vi "运维调试_总磷.vi"() -> ()   [LabVIEW 2016, in "斯坦道总磷.lvlib"]
uses:
  <vilib>/Utility/miscctls.llb/LVPointTypeDef.ctl
  <vilib>/Utility/config.llb/NI_LVConfig.lvlib
  <vilib>/ptbypt/NI_PtbyPt.lvlib
panel:
  out "二级权限":bool
  out "一级权限":bool
  out "输入密码":u32
  out "权限锁":bool
  in  "流程固件":bool
  in  "仪器参数设置":bool
  in  "量程参数读取":T1
  in  "模块启用":bool
  in  "串口设置":bool
  in  "公式一键写入":bool
  in  "流程路径":path=path "C:/Users/STD/Documents/斯坦道流程文件/流程.xml"
  in  "曲线模型":cluster{"X^2":dbl, "X":dbl, "B":dbl}(xcontrol)
  out "字符串":string
  in  "质控参数设置":bool
  in  "总磷自动测试量程配置":T2
  out "温度2":sgl
  out "温度1":sgl
  out "ADC":sgl
  out "固件版本号":string
  in  "数组":string[](array[string])
  in  "量程切换阈值写入":bool
  in  "量程切换阈值读取":bool
  in  "参数下拉列表":enum16{"总磷", "总氮"}(ring)
  in  "量程下拉列表":enum16{"低量程", "高量程"}(ring)
  in  "测量模式下拉列表":enum16{"水样测量", "零点核查", "跨度核查", "标样核查", "加标回收"}(ring)
  in  "公式":cluster{"X^2":dbl, "X":dbl, "b":dbl}
  in  "写公式":bool
  in  "读公式":bool
  in  "返回":bool
  in  "设置":bool
  out "序列号":string="序列号"
  out "测量数据":T3(xcontrol)
  out "集成报警信息":string
  out "定时启动":bool
  out "总磷总氮运行状态":T4(xcontrol)
  in  "停止":bool
  in  "手动启动":bool
  in  "单步测试":bool
  in  "总磷氨氮调试":u16[](xcontrol)
  out "F3":sgl format="%#.6f"
  out "F2":sgl format="%#.6f"
  out "F1":sgl format="%#.6f"
  out "F0":sgl format="%#.6f"
  out "多列列表框":i32(listbox)
  # "参数设置"
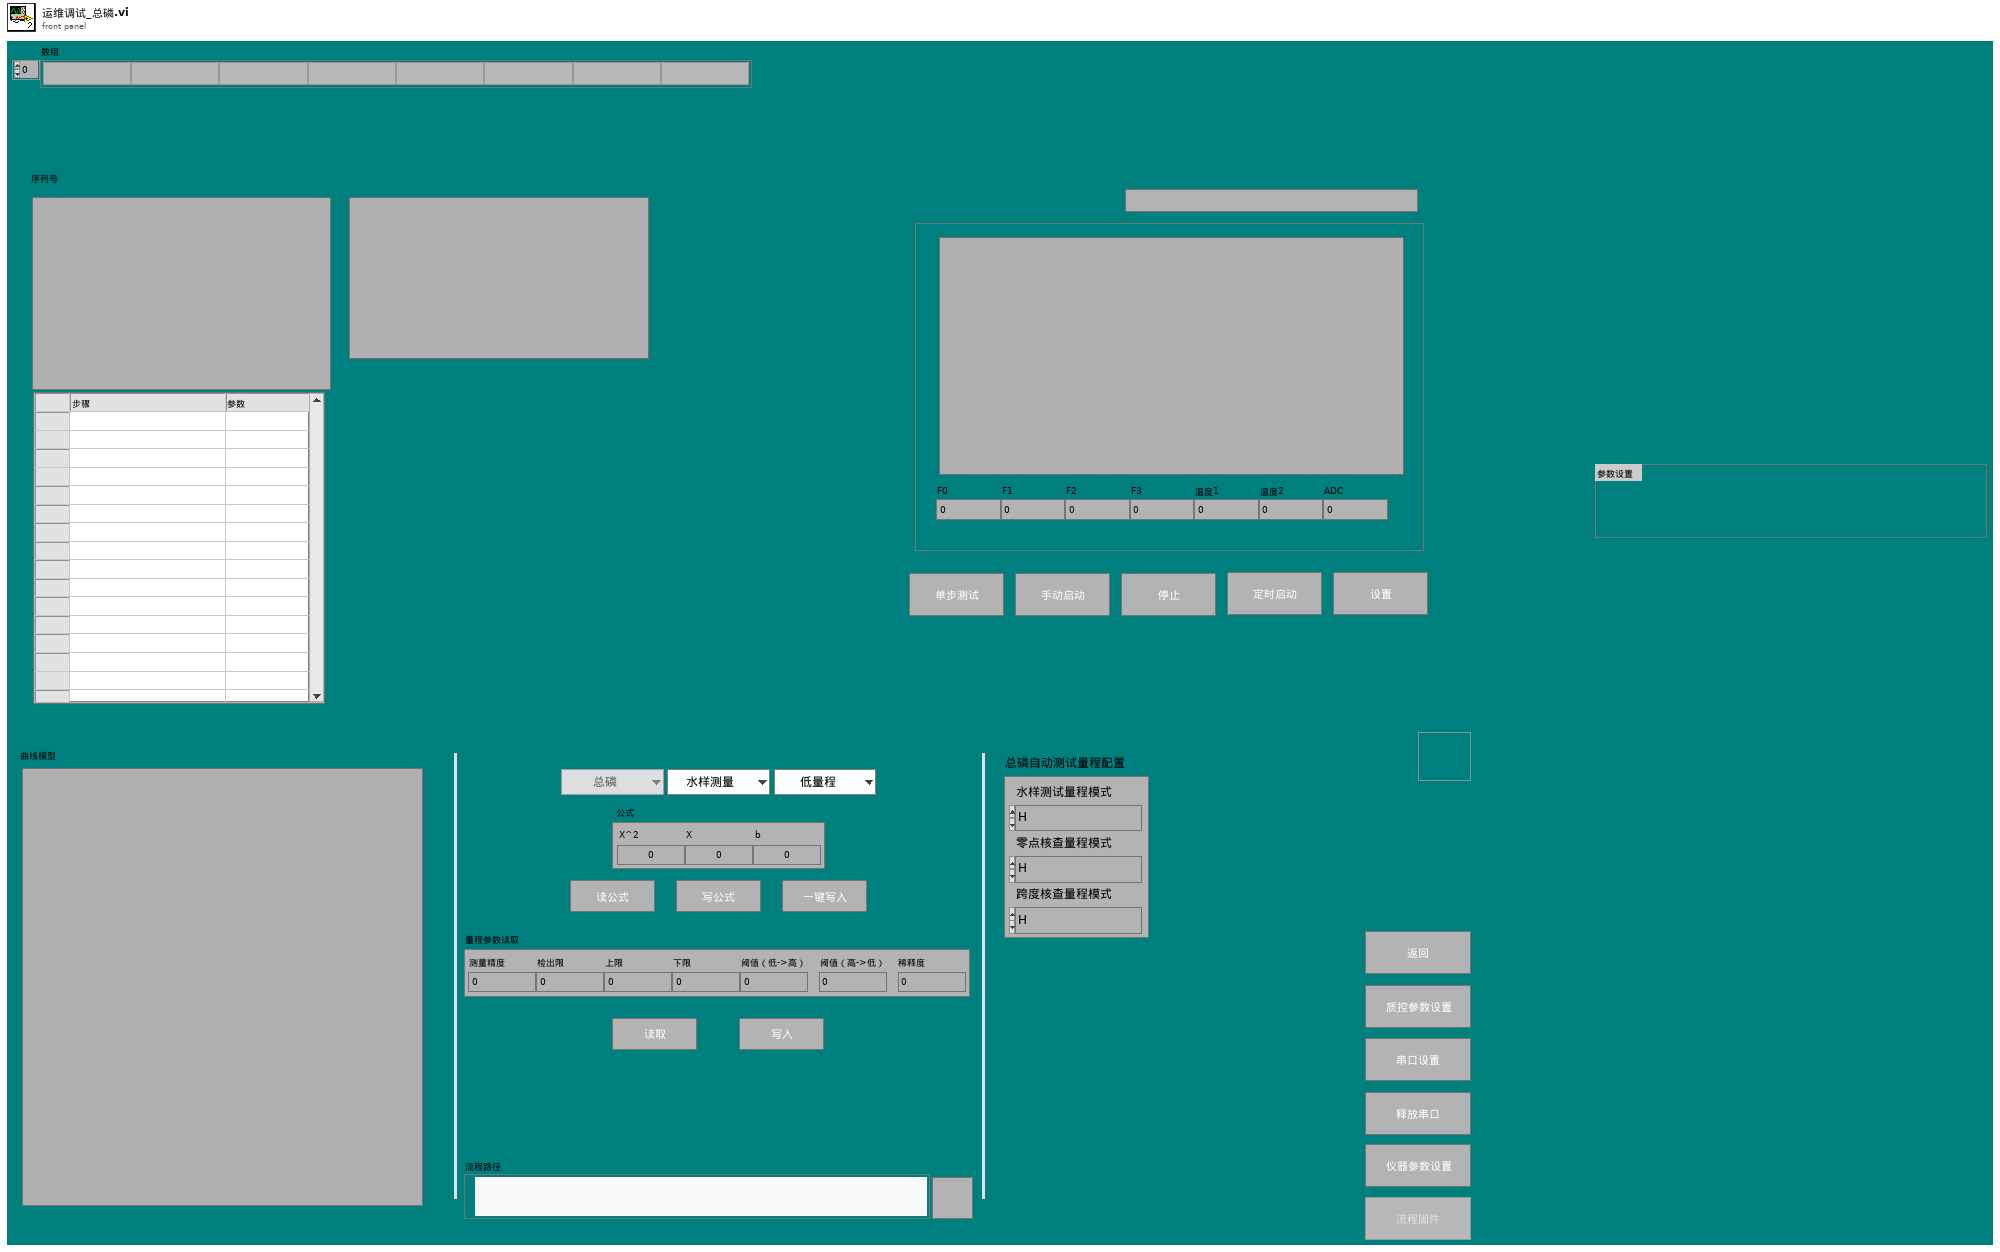
[diagram p1: front panel]
types:
  T1 = cluster{"测量精度":dbl, "检出限":dbl, "上限":dbl, "下限":dbl, "阈值（低->高）":dbl, "阈值（高->低）":dbl, "稀释度":dbl}
  T2 = cluster{"水样测试量程模式":enum16{"H", "L", "AUTO"}, "空白核查量程模式":enum16{"H", "L", "AUTO"}, "跨度核查量程模式":enum16{"H", "L", "AUTO"}}
  T3 = cluster{"flowid":u16, "测量精度":u16, "测量数据区":cluster{"因子编码":u32, "单位":u16, "标样参考值":sgl, "水样数据时间":timestamp, "水样实测值":sgl, "水样数据标识":string, "标样数据时间":timestamp, "标样实测值":sgl, "标样数据标识":string, "空白数据时间":timestamp, "空白实测值":sgl, "空白数据标识":string, "零点核查数据时间":timestamp, "零点核查实测值":sgl, "零点核查数据标识":string, "跨度核查数据时间":timestamp, "跨度核查实测值":sgl, "跨度核查数据标识":string, "加标回收数据时间":timestamp, "加标回收实测值":sgl, "加标回收数据标识":string, "平行样数据时间":timestamp, "平行样实测值":sgl, "平行样数据标识":string, "F0":sgl, "F1":sgl, "F2":sgl, "F3":sgl, "F4":sgl, "F5":sgl, "F6":sgl, "F7":sgl, "温度":sgl, "湿度":sgl, "X值":sgl, "fidrange":sgl}}
  T4 = cluster{"系统时间":timestamp, "工作状态":enum16{"空闲", "水样测试", "标样核查", "零点核查", "跨度核查", "空白测试", "平行样测试", "加标回收", "空白校准", "标样校准", "初始化（清洗）"}, "测量模式":enum16{"待机", "连续模式", "周期模式", "定点模式", "受控模式", "手动模式"}, "告警代码":u16, "故障代码":u16, "日志代码":u16, "软件版本":u16, "F0":sgl, "F1":sgl, "F2":sgl, "F3":sgl, "T":sgl, "H":sgl, "id":u16, "flowid":u16, "量程":u16, "总磷控温温度1":sgl, "营养盐控温温度2":sgl, "ADC":sgl}
  T5 = enum16{"启动测量", "标样核查", "零点核查", "跨度核查", "空白测试", "平行样测试", "加标回收", "空白校准", "标样校准", "初始化（清洗）", "停止测试", "仪器重启", "校时", "模式设置", "测量间隔设置"}
  T6 = cluster{"控制命令":enum16{"启动测量", "标样核查", "零点核查", "跨度核查", "空白测试", "平行样测试", "加标回收", "空白校准", "标样校准", "初始化（清洗）", "停止测试", "仪器重启", "校时", "模式设置", "测量间隔设置"}, "周期设置类型":enum16{"定点启动", "间隔启动"}, "定时功能启用":bool, "定时间隔":dbl, "24H周期设置":bool[], "零点核查时间":u16, "跨度核查时间":u16, "质控频次":enum16{"关闭", "每天", "星期一", "星期二", "星期三", "星期四", "星期五", "星期六", "星期日"}}
  T7 = enum16{"关闭", "每天", "星期一", "星期二", "星期三", "星期四", "星期五", "星期六", "星期日"}
  T8 = typedef "LVDateTimeRec.ctl" = cluster{"秒数的小数部分":dbl, "秒":i32, "分":i32, "时":i32, "日":i32, "月":i32, "年":i32, "天数（周）":i32, "天数（年）":i32, "DST":i32}
  T9 = enum16{"空闲", "水样测试", "标样核查", "零点核查", "跨度核查", "空白测试", "平行样测试", "加标回收", "空白校准", "标样校准", "初始化（清洗）"}
  T10 = enum32{"Bad", "Idle", "Run top level", "Running"}
  T11 = typedef "LVPointTypeDef.ctl" = cluster{"Horizontal":i16, "Vertical":i16}
  T12 = cluster{"因子编码":u32, "单位":u16, "标样参考值":sgl, "水样数据时间":timestamp, "水样实测值":sgl, "水样数据标识":string, "标样数据时间":timestamp, "标样实测值":sgl, "标样数据标识":string, "空白数据时间":timestamp, "空白实测值":sgl, "空白数据标识":string, "零点核查数据时间":timestamp, "零点核查实测值":sgl, "零点核查数据标识":string, "跨度核查数据时间":timestamp, "跨度核查实测值":sgl, "跨度核查数据标识":string, "加标回收数据时间":timestamp, "加标回收实测值":sgl, "加标回收数据标识":string, "平行样数据时间":timestamp, "平行样实测值":sgl, "平行样数据标识":string, "F0":sgl, "F1":sgl, "F2":sgl, "F3":sgl, "F4":sgl, "F5":sgl, "F6":sgl, "F7":sgl, "温度":sgl, "湿度":sgl, "X值":sgl, "fidrange":u16}
  T13 = typedef "NI_LVConfig.lvlib/Config Data RefNum.ctl" = refnum<k1>
  T14 = enum8{"Enabled", "Disabled", "Disabled and Grayed Out"}
  T15 = cluster{"启动模式":enum16{"跨度核查", "水样测量", "空白核查", "标样核查", "加标回收"}, "启动参数":u16, "量程":enum16{"低量程", "高量程"}}
  T16 = cluster{"时间标识":timestamp, "设备":string, "日志信息":string, "流程参数":string}
  T17 = cluster{"时间标识":timestamp, "设备":string, "日志信息":string}
  T18 = typedef "LVRowAndColumnUnsignedTypeDef.ctl" = cluster{"Row":u32, "Column":u32}
  T19 = cluster{"参数下拉列表":enum16{"总磷", "总氮"}, "测量模式下拉列表":enum16{"水样测量", "零点核查", "跨度核查", "标样核查", "加标回收"}, "量程下拉列表":enum16{"低量程", "高量程"}}
  T20 = cluster{"站号":u16, "量程切换":enum32{"H", "L", "AUTO"}, "控制命令":enum16{"启动测量", "标样核查", "零点核查", "跨度核查", "空白测试", "平行样测试", "加标回收", "空白校准", "标样校准", "初始化（清洗）", "停止测试", "仪器重启", "校时", "模式设置", "测量间隔设置"}, "模式设置":enum16{"待机", "连续模式", "周期模式", "定点模式", "受控模式", "手动模式"}, "测量间隔":u16}
  T21 = cluster{"总磷跨度值":dbl, "总磷零点标准液浓度":dbl, "总磷跨度标准液浓度":dbl, "总磷标准液标准浓度":dbl}
  T22 = cluster{"确定":bool, "总磷跨度值":dbl, "总磷零点标准液浓度":dbl, "总磷跨度标准液浓度":dbl, "总磷标准液标准浓度":dbl}
  T23 = cluster{"测量量程":dbl, "测量精度":dbl, "测量间隔":dbl, "消解温度":dbl, "消解时长":dbl, "空白校准时间":timestamp, "曲线截距":dbl, "曲线斜率":dbl, "测量检出限":dbl, "测量信号值":dbl, "线性相关系数":dbl, "二次多项式系数":dbl, "标样校准时间":timestamp, "单位":u16}
  T24 = cluster{"确定":bool, "测量量程":dbl, "测量精度":dbl, "测量间隔":dbl, "消解温度":dbl, "消解时长":dbl, "空白校准时间":timestamp, "曲线截距":dbl, "曲线斜率":dbl, "测量检出限":dbl, "测量信号值":dbl, "线性相关系数":dbl, "二次多项式系数":dbl, "标样校准时间":timestamp, "单位":u16}
  T25 = cluster{"控制命令":enum16{"启动测量", "标样核查", "零点核查", "跨度核查", "空白测试", "平行样测试", "加标回收", "空白校准", "标样校准", "初始化（清洗）", "停止测试", "仪器重启", "校时", "模式设置", "测量间隔设置"}, "周期设置类型":enum16{"定点启动", "间隔启动"}, "定时功能启用":bool, "定时间隔":dbl, "24H周期设置":bool[], "空白核查时间":u16, "跨度核查时间":u16, "质控频次":enum16{"关闭", "每天", "星期一", "星期二", "星期三", "星期四", "星期五", "星期六", "星期日"}}
  T26 = cluster{"测量精度":u16, "检出限":dbl, "上限":dbl, "下限":dbl, "阈值（低->高）":dbl, "阈值（高->低）":dbl, "稀释度":dbl}
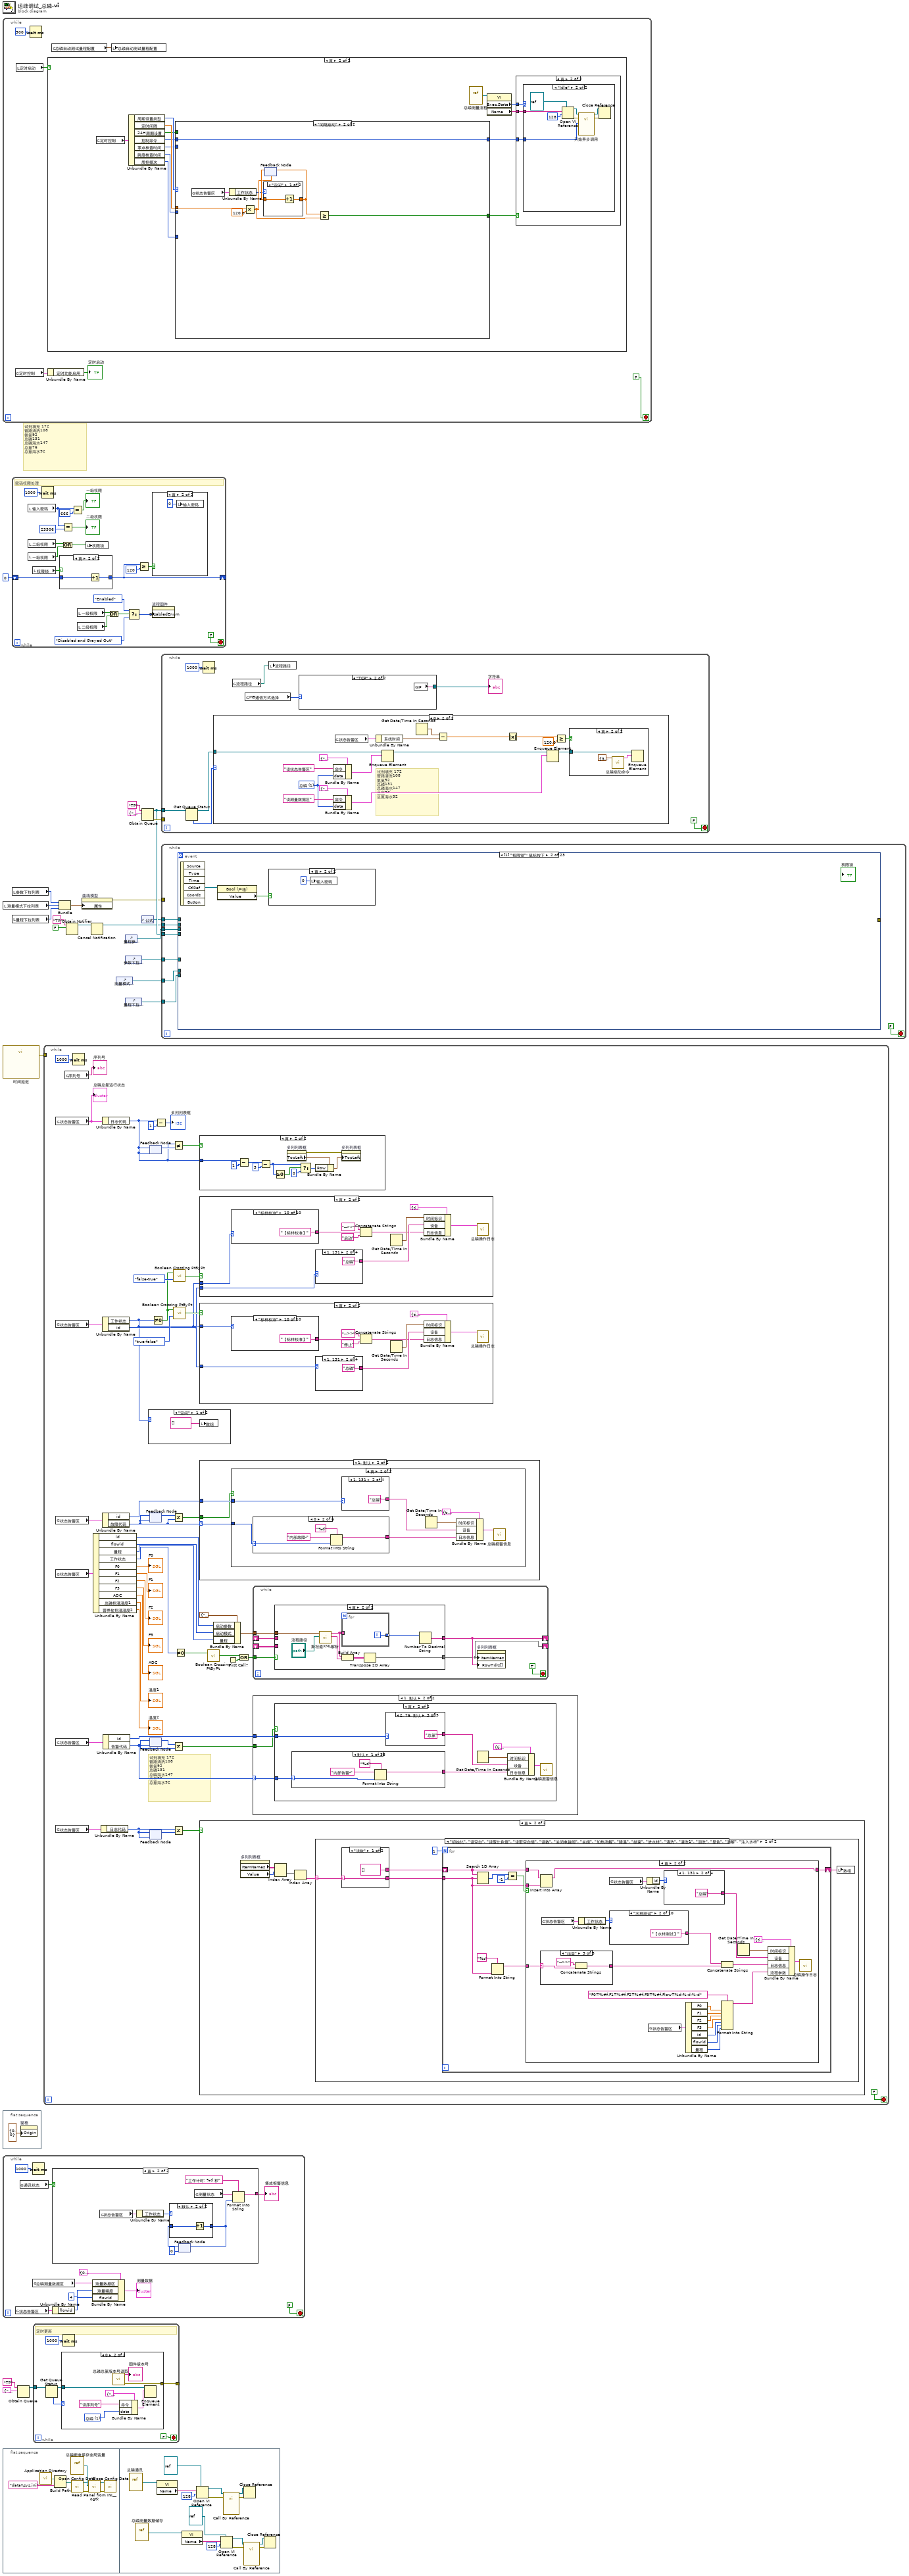
[diagram p0: block diagram]
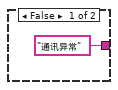
[diagram p5: hidden frame]
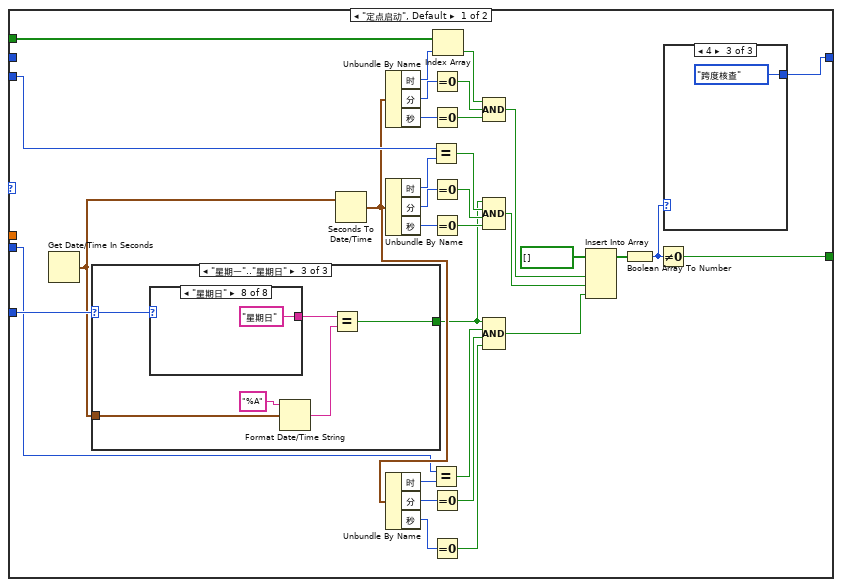
[diagram p8: hidden frame]
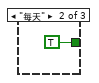
[diagram p10: hidden frame]
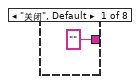
[diagram p11: hidden frame]
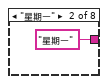
[diagram p12: hidden frame]
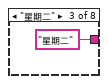
[diagram p13: hidden frame]
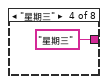
[diagram p14: hidden frame]
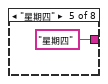
[diagram p15: hidden frame]
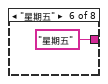
[diagram p16: hidden frame]
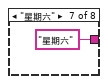
[diagram p17: hidden frame]
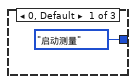
[diagram p18: hidden frame]
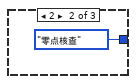
[diagram p19: hidden frame]
diagram:
  # "试剂填充 172 \n管路清洗108\n氨氮92\n总磷131\n总磷海水147\n总氮76\n总氮海水92"
  n1 = while {
    stop <- FALSE stop-if-true
    n2 = global read "总磷断电保存全局变量.vi" "定时控制"() -> (w25:T6)
    n3 = local read "定时启动"() -> (w27:bool)
    n4 = Wait (ms)(milliseconds to wait=u32 500 ("等待时间（毫秒）")) -> ()  [unwired: 1 out]
    n5 = case shown="真" w27 {
      frame False {
      }
      frame True {
        n6 = global read "总磷断电保存全局变量.vi" "定时控制"() -> (w42:T6)
        n7 = Unbundle By Name(w42) -> ("周期设置类型"=w39:enum16{"定点启动", "间隔启动"}, "定时间隔"=w37:dbl, "24H周期设置"=w36:bool[], "控制命令"=w34:T5, "零点核查时间"=w33:u16, "跨度核查时间"=w32:u16, "质控频次"=w31:T7)
        n8 = case shown="\"间隔启动\"" w39 {
          tunnel: w37 -> [_ w100]
          tunnel: w36 -> [w66 _]
          tunnel: [w44 w98] -> w30
          tunnel: w34 -> [_ w96]
          tunnel: [w70 w96] -> w35
          tunnel: w31 -> [w69 _]
          tunnel: w33 -> [w62 _]
          tunnel: w32 -> [w51 _]
          frame "定点启动", Default {
            n9 = Get Date/Time In Seconds() -> (seconds since 1Jan1904=w68:timestamp)
            n10 = case shown="\"星期一\"..\"星期日\"" w69 {
              selector: w69 -> [_ _ w80]
              tunnel: w68 -> [_ _ w81]
              tunnel: [_ TRUE w77] -> w50
              frame "关闭", Default {
              }
              frame "每天" {
              }
              frame "星期一".."星期日" {
                n11 = case shown="\"星期日\"" w80 {
                  tunnel: ["" ("时间格式字符串(%c)") "星期一" ("时间格式字符串(%c)") "星期二" ("时间格式字符串(%c)") "星期三" ("时间格式字符串(%c)") "星期四" ("时间格式字符串(%c)") "星期五" ("时间格式字符串(%c)") "星期六" ("时间格式字符串(%c)") "星期日" ("时间格式字符串(%c)")] -> w79
                  frame "关闭", Default {
                  }
                  frame "星期一" {
                  }
                  frame "星期二" {
                  }
                  frame "星期三" {
                  }
                  frame "星期四" {
                  }
                  frame "星期五" {
                  }
                  frame "星期六" {
                  }
                  frame "星期日" {
                  }
                }
                n12 = Format Date/Time String(time format string (%c)="%A" ("时间格式字符串(%c)"), seconds (now)=w81) -> (date/time string=w78:string)  [unwired: 1 in]
                n13 = Equal?(x=w79, y=w78) -> (x = y?=w77:bool)
              }
            }
            n14 = Seconds To Date/Time(time stamp (now)=w68) -> (date time rec=w52:T8)  [unwired: 1 in]
            n15 = Unbundle By Name(w52) -> ("时"=w75:i32, "分"=w73:i32, "秒"=w74:i32)
            n16 = Unbundle By Name(w52) -> ("时"=w63:i32, "分"=w65:i32, "秒"=w64:i32)
            n17 = Unbundle By Name(w52) -> ("时"=w55:i32, "分"=w53:i32, "秒"=w54:i32)
            n18 = Equal?(x=w62, y=w63) -> (x = y?=w61:bool)
            n19 = Equal?(x=w51, y=w55) -> (x = y?=w56:bool)
            n20 = Equal To 0?(x=w73) -> (x = 0?=w72:bool)
            n21 = Equal To 0?(x=w74) -> (x = 0?=w71:bool)
            n22 = Equal To 0?(x=w65) -> (x = 0?=w60:bool)
            n23 = Equal To 0?(x=w64) -> (x = 0?=w59:bool)
            n24 = Equal To 0?(x=w53) -> (x = 0?=w57:bool)
            n25 = Equal To 0?(x=w54) -> (x = 0?=w58:bool)
            n26 = Index Array(array=w66, index=w75) -> (element=w67:bool)
            n27 = Compound Arithmetic op=AND ("复合运算")(w67, w72, w71) -> (w48:bool)
            n28 = Compound Arithmetic op=AND ("复合运算")(w50, w61, w60, w59) -> (w47:bool)
            n29 = Compound Arithmetic op=AND ("复合运算")(w50, w56, w57, w58) -> (w46:bool)
            n30 = Insert Into Array(array=bool[] [], new element #1=w48, new element #2=w47, new element #3=w46) -> (w45:bool[])  [unwired: 1 in]
            n31 = Boolean Array To Number(Boolean array=w45) -> (number=w43:u32)
            n32 = Not Equal To 0?(x=w43) -> (x != 0?=w44:bool)
            n33 = case shown="4" w43 {
              tunnel: [T5."启动测量" ("控制命令") T5."零点核查" ("控制命令") T5."跨度核查" ("控制命令")] -> w70
              frame 0, Default {
              }
              frame 2 {
              }
              frame 4 {
              }
            }
          }
          frame "间隔启动" {
            n34 = global read "VAR总磷全局变量.vi" "状态告警区"() -> (w95:T4)
            n35 = Unbundle By Name(w95) -> ("工作状态"=w94:T9)
            n36 = Multiply(x=w100, y=120.0) -> (x*y=w97:dbl)
            n37 = feedback #1(w97) -> (w102:dbl)
            n38 = case shown="\"空闲\"" w94 {
              tunnel: w102 -> [w104 _]
              tunnel: [w103 _] -> w101
              frame "空闲" {
                n39 = Increment(x=w104) -> (x+1=w103:dbl)
              }
              frame "水样测试", Default {
              }
            }
            n40 = feedback-in #1(w101) -> ()
            n41 = Greater Or Equal?(x=w101, y=w97) -> (x >= y?=w98:bool)
          }
        }
        n42 = vi-ref "总磷测量流程.vi"() -> (w41:refnum<vi>)
        n43 = property class="VI"(reference=w41) -> ("Exec.State"=w38:T10, "Name"=w40:string)  [unwired: 1 in, 2 out]
        n44 = case shown="真" w30 {
          tunnel: w40 -> [_ w107]
          tunnel: w35 -> [_ w106]
          tunnel: w38 -> [_ w105]
          frame False {
          }
          frame True {
            n45 = case shown="\"Idle\"" w105 {
              tunnel: w107 -> [_ w111]
              tunnel: w106 -> [_ w109]
              frame "Bad", Default {
              }
              frame "Idle" {
                n46 = Open VI Reference(type specifier VI Refnum (for type only)=refnum<vi> refnum, vi path=w111, options=128 ("选项")) -> (vi reference=w112:refnum<vi>, error out=w113:errorcluster)  [unwired: 3 in]
                n47 = call-by-ref "开始异步调用"(reference=w112, error in=w113, "控制命令"=w109) -> (reference out=w114:refnum<vi>, error out=w115:errorcluster)  [unwired: 11 in]
                n48 = Close Reference(reference=w114, error in (no error)=w115) -> ()  [unwired: 1 out]
              }
            }
          }
        }
      }
    }
    n49 = Unbundle By Name(w25) -> ("定时功能启用"=→"定时启动":bool)
    n50 = global read "总磷断电保存全局变量.vi" "总磷自动测试量程配置"() -> (w26:T2)
    n51 = local write "总磷自动测试量程配置"(w26) -> ()
  }
  n52 = local read "测量模式下拉列表"() -> (w3:enum16{"水样测量", "零点核查", "跨度核查", "标样核查", "加标回收"})
  n53 = call "时间延迟"() -> ("error out"=w15:errorcluster)  [unwired: 11 in]
  n54 = flat-sequence {
    frame #0 {
      n55 = property on="窗格" class="Pane"("Origin"=T11 {"Horizontal"=0, "Vertical"=0} ("原点")) -> ()  [unwired: 2 in, 2 out]
    }
  }
  n56 = while {
    stop <- FALSE stop-if-true
    n57 = global read "VAR总磷全局变量.vi" "状态告警区"() -> (w122:T4)
    n58 = global read "VAR总磷全局变量.vi" "通讯状态"() -> (w124:bool)
    n59 = Wait (ms)(milliseconds to wait=u32 1000 ("等待时间（毫秒）")) -> ()  [unwired: 1 out]
    n60 = global read "VAR总磷全局变量.vi" "总磷测量数据区"() -> (w119:T12)
    n61 = case shown="真" w124 {
      tunnel: ["通讯异常" ("集成报警信息") w129] -> w123
      frame False {
      }
      frame True {
        n62 = global read "VAR总磷全局变量.vi" "状态告警区"() -> (w135:T4)
        n63 = Unbundle By Name(w135) -> ("工作状态"=w134:T9)
        n64 = feedback #2(0) -> (w132:i32)
        n65 = case shown="默认" w134 {
          tunnel: w132 -> [_ w137]
          tunnel: [_ w136] -> w130
          frame "空闲" {
          }
          frame Default {
            n66 = Increment(x=w137) -> (x+1=w136:i32)
          }
        }
        n67 = feedback-in #2(w130) -> ()
        n68 = global read "VAR总磷全局变量.vi" "测量状态"() -> (w128:string)
        n69 = Format Into String(format string="工作计时: %d 秒" ("格式字符串"), initial string=w128, w130) -> (resulting string=w129:string)  [unwired: 1 in, 1 out]
      }
    }
    "集成报警信息" <- w123
    n70 = Unbundle By Name(w122) -> ("flowid"=w121:u16)
    n71 = Bundle By Name(cluster=T3 {"flowid"=0, "测量精度"=0, "测量数据区"={"因子编码"=0, "单位"=0, "标样参考值"=0.0, "水样数据时间"=timestamp(0 s since 1904-01-01), "水样实测值"=0.0, "水样数据标识"="", "标样数据时间"=timestamp(0 s since 1904-01-01), "标样实测值"=0.0, "标样数据标识"="", "空白数据时间"=timestamp(0 s since 1904-01-01), "空白实测值"=0.0, "空白数据标识"="", "零点核查数据时间"=timestamp(0 s since 1904-01-01), "零点核查实测值"=0.0, "零点核查数据标识"="", "跨度核查数据时间"=timestamp(0 s since 1904-01-01), "跨度核查实测值"=0.0, "跨度核查数据标识"="", "加标回收数据时间"=timestamp(0 s since 1904-01-01), "加标回收实测值"=0.0, "加标回收数据标识"="", "平行样数据时间"=timestamp(0 s since 1904-01-01), "平行样实测值"=0.0, "平行样数据标识"="", "F0"=0.0, "F1"=0.0, "F2"=0.0, "F3"=0.0, "F4"=0.0, "F5"=0.0, "F6"=0.0, "F7"=0.0, "温度"=0.0, "湿度"=0.0, "X值"=0.0, "fidrange"=0.0}} ("测量数据"), "测量数据区"=w119, "测量精度"=u16 4, "flowid"=w121) -> (→"测量数据":T3)
  }
  n72 = flat-sequence {
    frame #0 {
      n73 = call <vilib>:"Application Directory.vi"() -> ("Application Directory"=w145:path)
      n74 = Build Path(base path=w145, name or relative path="data\\sys.ini" ("名称或相对路径")) -> (appended path=w143:path)
      n75 = vi-ref "总磷断电保存全局变量.vi"() -> (w141:refnum<vi>)
      n76 = call <vilib>:"Open Config Data.vi"("configuration file path"=w143) -> ("error out"=w139:errorcluster, "refnum"=w142:T13)  [unwired: 8 in, 1 out]
      n77 = call <userlib>:"Read Panel from INI__ogtk.vi"("error in (no error)"=w139, "VI ref"=w141, "refnum"=w142) -> ("error out"=w138:errorcluster, "refnum out"=w140:T13)  [unwired: 7 in]
      n78 = call <vilib>:"Close Config Data.vi"("error in (no error)"=w138, "refnum"=w140) -> ()  [unwired: 8 in, 2 out]
    }
    frame #1 {
      n79 = vi-ref "总磷通讯.vi"() -> (w161:refnum<vi>)
      n80 = vi-ref "总磷测量数据储存.vi"() -> (w153:refnum<vi>)
      n81 = property class="VI"(reference=w161) -> ("Name"=w160:string)  [unwired: 1 in, 2 out]
      n82 = property class="VI"(reference=w153) -> ("Name"=w146:string)  [unwired: 1 in, 2 out]
      n83 = Open VI Reference(type specifier VI Refnum (for type only)=refnum<vi> refnum, vi path=w160, options=128 ("选项")) -> (vi reference=w158:refnum<vi>, error out=w156:errorcluster)  [unwired: 3 in]
      n84 = Open VI Reference(type specifier VI Refnum (for type only)=refnum<vi> refnum, vi path=w146, options=128 ("选项")) -> (vi reference=w148:refnum<vi>, error out=w150:errorcluster)  [unwired: 3 in]
      n85 = call-by-ref "?"(reference=w158, error in=w156) -> (reference out=w154:refnum<vi>, error out=w155:errorcluster)  [unwired: 12 in]
      n86 = Close Reference(reference=w154, error in (no error)=w155) -> ()  [unwired: 1 out]
      n87 = call-by-ref "?"(reference=w148, error in=w150) -> (reference out=w152:refnum<vi>, error out=w151:errorcluster)  [unwired: 12 in]
      n88 = Close Reference(reference=w152, error in (no error)=w151) -> ()  [unwired: 1 out]
    }
  }
  n89 = while {
    shift-right: [w164] -> _
    shift-left: u32 0 ("等待时间（毫秒）") -> [w165]
    stop <- FALSE stop-if-true
    # "密码权限处理"
    n90 = local read "输入密码"() -> (w176:u32)
    n91 = local read "二级权限"() -> (w172:bool)
    n92 = local read "一级权限"() -> (w178:bool)
    n93 = local read "权限锁"() -> (w166:bool)
    n94 = Wait (ms)(milliseconds to wait=u32 1000 ("等待时间（毫秒）")) -> ()  [unwired: 1 out]
    n95 = case shown="真" w166 {
      tunnel: w165 -> [_ w185]
      tunnel: [_ w184] -> w164
      frame False {
      }
      frame True {
        n96 = Increment(x=w185) -> (x+1=w184:u32)
      }
    }
    n97 = Or(x=w172, y=w178) -> (x .or. y?=w173:bool)
    n98 = Equal?(x=w176, y=u32 23506) -> (x = y?=→"二级权限":bool)
    n99 = Equal?(x=w176, y=u32 666) -> (x = y?=→"一级权限":bool)
    n100 = local read "一级权限"() -> (w177:bool)
    n101 = local read "二级权限"() -> (w167:bool)
    n102 = local write "权限锁"(w173) -> ()
    n103 = Or(x=w177, y=w167) -> (x .or. y?=w168:bool)
    n104 = Select(t=T14."Enabled" ("禁用"), s=w168, f=T14."Disabled and Grayed Out" ("禁用")) -> (s? t:f=w169:T14)
    n105 = Greater Or Equal?(x=w164, y=u32 120) -> (x >= y?=w162:bool)
    n106 = case shown="真" w162 {
      frame False {
      }
      frame True {
        n107 = local write "输入密码"(u32 0 ("输入密码")) -> ()
      }
    }
    n108 = property on="流程固件" class="Bool"("DisabledEnum"=w169) -> ()  [unwired: 2 in, 2 out]
  }
  n109 = local read "参数下拉列表"() -> (w4:enum16{"总磷", "总氮"})
  n110 = local read "量程下拉列表"() -> (w2:enum16{"低量程", "高量程"})
  n111 = Obtain Queue(name (unnamed)="TP" ("名称（未命名）"), element data type=cluster{"命令":string, "data":variant} {"命令"="", "data"=variant}) -> (queue out=w12:refnum<queue>)  [unwired: 3 in, 2 out]
  n112 = while {
    tunnel: w12 -> [w190]
    tunnel: [w188] -> _
    stop <- FALSE stop-if-true
    # "定时更新"
    n113 = Get Queue Status(queue=w190) -> (queue out=w187:refnum<queue>, # elements in queue=w186:i32)  [unwired: 2 in, 6 out]
    n114 = case shown="0" w186 {
      tunnel: w187 -> [_ w195]
      tunnel: [_ w192] -> w188
      frame Default {
      }
      frame 0 {
        w196 = u16 1 items=["总磷"=1, "氨氮"=3] ("站号")
        n115 = call "总磷总氮版本号读取.vi"() -> ("error out"=w192:errorcluster, "固件版本号"=→"固件版本号":string)  [unwired: 10 in]
        n116 = Bundle By Name(cluster=cluster{"命令":string, "data":variant} {"命令"="", "data"=variant} ("元素"), "命令"="读序列号", "data"=w196) -> (w194:cluster{"命令":string, "data":variant})
        n117 = Enqueue Element(queue=w195, element=w194) -> ()  [unwired: 2 in, 3 out]
      }
    }
    n118 = Wait (ms)(milliseconds to wait=u32 1000 ("等待时间（毫秒）")) -> ()  [unwired: 1 out]
  }
  n119 = while {
    tunnel: w15 -> [_]
    stop <- FALSE stop-if-true
    # "试剂填充 172 \n管路清洗108\n氨氮92\n总磷131\n总磷海水147\n总氮76\n总氮海水92"
    n120 = global read "VAR总磷全局变量.vi" "状态告警区"() -> (w232:T4)
    "总磷总氮运行状态" <- w232
    n121 = global read "VAR总磷全局变量.vi" "状态告警区"() -> (w219:T4)
    n122 = global read "VAR总磷全局变量.vi" "状态告警区"() -> (w224:T4)
    n123 = global read "VAR总磷全局变量.vi" "状态告警区"() -> (w240:T4)
    n124 = global read "VAR总磷全局变量.vi" "状态告警区"() -> (w229:T4)
    n125 = global read "VAR总磷全局变量.vi" "状态告警区"() -> (w217:T4)
    n126 = global read "VAR总磷全局变量.vi" "序列号"() -> (→"序列号":string)
    n127 = Wait (ms)(milliseconds to wait=u32 1000 ("等待时间（毫秒）")) -> ()  [unwired: 1 out]
    n128 = Unbundle By Name(w240) -> ("id"=w237:u16, "flowid"=w239:u16, "量程"=w238:u16, "工作状态"=w207:T9, "F0"=→"F0":sgl, "F1"=→"F1":sgl, "F2"=→"F2":sgl, "F3"=→"F3":sgl, "ADC"=→"ADC":sgl, "总磷控温温度1"=→"温度1":sgl, "营养盐控温温度2"=→"温度2":sgl)
    n129 = Unbundle By Name(w217) -> ("日志代码"=w216:u16)
    n130 = Unbundle By Name(w232) -> ("日志代码"=w213:u16)
    n131 = Unbundle By Name(w219) -> ("工作状态"=w199:T9, "id"=w200:u16)
    n132 = Unbundle By Name(w224) -> ("id"=w223:u16, "故障代码"=w220:u16)
    n133 = Unbundle By Name(w229) -> ("id"=w228:u16, "告警代码"=w225:u16)
    n134 = case shown="\"空闲\"" w199 {
      frame "空闲" {
        n135 = local write "数组"(string[] [] ("数组")) -> ()
      }
      frame "水样测试", Default {
      }
    }
    n136 = feedback-in #3(w213) -> ()
    n137 = feedback #3(w213) -> (w245:u16)
    n138 = feedback #4(w220) -> (w221:u16)
    n139 = feedback-in #4(w220) -> ()
    n140 = feedback #5(w225) -> (w226:u16)
    n141 = feedback-in #5(w225) -> ()
    n142 = feedback #6(w216) -> (w218:u16)
    n143 = feedback-in #6(w216) -> ()
    n144 = Not Equal To 0?(x=w199) -> (x != 0?=w202:bool)
    n145 = Subtract(x=w213, y=1) -> (x-y=→"多列列表框":i32)
    n146 = Not Equal?(x=w213, y=w245) -> (x != y?=w244:bool)
    n147 = Not Equal?(x=w221, y=w220) -> (x != y?=w222:bool)
    n148 = Not Equal?(x=w226, y=w225) -> (x != y?=w227:bool)
    n149 = Not Equal?(x=w216, y=w218) -> (x != y?=w215:bool)
    n150 = call <vilib>:"Boolean Crossing PtByPt.vi"("direction"=enum16{"either", "false-true", "true-false"}."false-true", "input"=w202) -> ("crossing"=w204:bool)  [unwired: 1 in]
    n151 = call <vilib>:"Boolean Crossing PtByPt.vi"("direction"=enum16{"either", "false-true", "true-false"}."true-false", "input"=w202) -> ("crossing"=w201:bool)  [unwired: 1 in]
    n152 = Not Equal To 0?(x=w207) -> (x != 0?=w242:bool)
    n153 = case shown="真" w244 {
      tunnel: w213 -> [_ w458]
      frame False {
      }
      frame True {
        n154 = Subtract(x=w458, y=1) -> (x-y=w456:i32)
        n155 = Subtract(x=w456, y=5) -> (x-y=w460:i32)
        n156 = Greater Or Equal To 0?(x=w460) -> (x >= 0?=w459:bool)
        n157 = property on="多列列表框" class="MCListbox (严格)"() -> (error out=w464:errorcluster, "TopLeft"=w465:T18)  [unwired: 2 in, 1 out]
        n158 = Select(t=w460, s=w459, f=0) -> (s? t:f=w461:i32)
        n159 = Bundle By Name(cluster=w465, "Row"=w461) -> (w466:T18)
        n160 = property on="多列列表框" class="MCListbox (严格)"(error in=w464, "TopLeft"=w466) -> ()  [unwired: 1 in, 2 out]
      }
    }
    n161 = case shown="真" w204 {
      tunnel: w199 -> [_ w279]
      tunnel: w200 -> [_ w275]
      frame False {
      }
      frame True {
        n162 = case shown="\"标样校准\"" w279 {
          tunnel: [_ "【水样测试】" ("字符串") "【标样核查】" ("字符串") "【零点核查】" ("字符串") "【跨度核查】" ("字符串") "【空白测试】" ("字符串") "【平行样测试】" ("字符串") "【加标回收】" ("字符串") "【空白校准】" ("字符串") "【标样校准】" ("字符串")] -> w273
          frame "空闲", Default {
          }
          frame "水样测试" {
          }
          frame "标样核查" {
          }
          frame "零点核查" {
          }
          frame "跨度核查" {
          }
          frame "空白测试" {
          }
          frame "平行样测试" {
          }
          frame "加标回收" {
          }
          frame "空白校准" {
          }
          frame "标样校准" {
          }
        }
        n163 = case shown="1, 131" w275 {
          tunnel: [_ "总磷" ("table输入") "氨氮" ("table输入") "总氮" ("table输入")] -> w274
          frame Default {
          }
          frame 1, 131 {
          }
          frame 3, 92 {
          }
          frame 2, 76 {
          }
        }
        n164 = Concatenate Strings("-->>" ("字符串"), w273, "启动" ("字符串")) -> (w270:string)
        n165 = Get Date/Time In Seconds() -> (seconds since 1Jan1904=w277:timestamp)
        n166 = Bundle By Name(cluster=T16 {"时间标识"=timestamp(0 s since 1904-01-01), "设备"="", "日志信息"="", "流程参数"=""} ("data in"), "时间标识"=w277, "设备"=w274, "日志信息"=w270) -> (w278:T16)
        n167 = call "总磷操作日志.vi"("data in"=w278) -> ()  [unwired: 11 in]
      }
    }
    n168 = case shown="真" w201 {
      tunnel: w199 -> [_ w257]
      tunnel: w200 -> [_ w253]
      frame False {
      }
      frame True {
        n169 = case shown="\"标样校准\"" w257 {
          tunnel: [_ "【水样测试】" ("字符串") "【标样核查】" ("字符串") "【零点核查】" ("字符串") "【跨度核查】" ("字符串") "【空白测试】" ("字符串") "【平行样测试】" ("字符串") "【加标回收】" ("字符串") "【空白校准】" ("字符串") "【标样校准】" ("字符串")] -> w251
          frame "空闲", Default {
          }
          frame "水样测试" {
          }
          frame "标样核查" {
          }
          frame "零点核查" {
          }
          frame "跨度核查" {
          }
          frame "空白测试" {
          }
          frame "平行样测试" {
          }
          frame "加标回收" {
          }
          frame "空白校准" {
          }
          frame "标样校准" {
          }
        }
        n170 = case shown="1, 131" w253 {
          tunnel: [_ "总磷" ("table输入") "氨氮" ("table输入") "总氮" ("table输入")] -> w252
          frame Default {
          }
          frame 1, 131 {
          }
          frame 3, 92 {
          }
          frame 2, 76 {
          }
        }
        n171 = Concatenate Strings("-->>" ("字符串"), w251, "停止" ("字符串")) -> (w248:string)
        n172 = Get Date/Time In Seconds() -> (seconds since 1Jan1904=w255:timestamp)
        n173 = Bundle By Name(cluster=T16 {"时间标识"=timestamp(0 s since 1904-01-01), "设备"="", "日志信息"="", "流程参数"=""} ("data in"), "时间标识"=w255, "设备"=w252, "日志信息"=w248) -> (w256:T16)
        n174 = call "总磷操作日志.vi"("data in"=w256) -> ()  [unwired: 11 in]
      }
    }
    n175 = case shown="1, 默认" w220 {
      selector: w220 -> [_ w360]
      tunnel: w223 -> [_ w361]
      tunnel: w222 -> [_ w359]
      frame 0 {
      }
      frame 1, Default {
        n176 = case shown="真" w359 {
          tunnel: w361 -> [_ w368]
          tunnel: w360 -> [_ w363]
          frame False {
          }
          frame True {
            n177 = case shown="0" w363 {
              selector: w363 -> [w370 w374 _ _ _ _]
              tunnel: [w369 w373 "电机故障" "温度故障" "通讯故障" "滴定故障"] -> w362
              frame Default {
                n178 = Format Into String(format string="%d" ("格式字符串"), initial string="未知" ("工作状态"), w370) -> (resulting string=w369:string)  [unwired: 1 in, 1 out]
              }
              frame 0 {
                n179 = Format Into String(format string="%d" ("格式字符串"), initial string="内部故障-" ("工作状态"), w374) -> (resulting string=w373:string)  [unwired: 1 in, 1 out]
              }
              frame 1 {
              }
              frame 2 {
              }
              frame 3 {
              }
              frame 4 {
              }
            }
            n180 = case shown="1, 131" w368 {
              tunnel: [_ "总磷" ("table输入") "氨氮" ("table输入") "总氮" ("table输入")] -> w364
              frame Default {
              }
              frame 1, 131 {
              }
              frame 3, 92 {
              }
              frame 2, 76 {
              }
            }
            n181 = Get Date/Time In Seconds() -> (seconds since 1Jan1904=w365:timestamp)
            n182 = Bundle By Name(cluster=T17 {"时间标识"=timestamp(0 s since 1904-01-01), "设备"="", "日志信息"=""} ("data in"), "时间标识"=w365, "设备"=w364, "日志信息"=w362) -> (w366:T17)
            n183 = call "总磷报警信息.vi"("data in"=w366) -> ()  [unwired: 10 in, 1 out]
          }
        }
      }
    }
    n184 = case shown="真" w215 {
      frame False {
      }
      frame True {
        n185 = property on="多列列表框" class="MCListbox (严格)"() -> ("ItemNames"=w295:string[][], "Value"=w296:i32)  [unwired: 2 in, 2 out]
        n186 = Index Array(array=w295, index (row)=w296) -> (element=w294:string[])  [unwired: 1 in]
        n187 = Index Array(array=w294) -> (element=w293:string)  [unwired: 1 in]
        n188 = case shown="\"初始化\", \"读空白\", \"读取比色值\", \"读取空白值\", \"读数\", \"关闭电磁阀\", \"关阀\", \"加热消解\", \"降温\", \"结束\", \"进水样\", \"清洗\", \"清洗1\", \"润洗\", \"显色\", \"消解\", \"注入水样\"" w293 {
          selector: w293 -> [_ w299]
          frame Default {
          }
          frame "初始化", "读空白", "读取比色值", "读取空白值", "读数", "关闭电磁阀", "关阀", "加热消解", "降温", "结束", "进水样", "清洗", "清洗1", "润洗", "显色", "消解", "注入水样" {
            n189 = case shown="\"读数\"" w299 {
              selector: w299 -> [w303 w305]
              tunnel: [w303 w305] -> w298
              tunnel: [string[] [] ("数组") "数组"] -> w297
              frame "读数" {
              }
              frame Default {
              }
            }
            n190 = for {
              N: 1 -> [_]
              tunnel: w298 -> [w307]
              shift-right: [w306] -> w300
              shift-left: w297 -> [w308]
              n191 = Search 1D Array(1D array=w308, element=w307) -> (index of element=w311:i32)  [unwired: 1 in]
              n192 = Format Into String(format string="%s" ("格式字符串"), w307) -> (resulting string=w312:string)  [unwired: 2 in, 1 out]
              n193 = Equal?(x=w311, y=-1) -> (x = y?=w309:bool)
              n194 = case shown="真" w309 {
                tunnel: w312 -> [_ w320]
                tunnel: w308 -> [w314 w324]
                tunnel: w307 -> [_ w323]
                tunnel: [w314 w322] -> w306
                frame False {
                }
                frame True {
                  n195 = Insert Into Array(array=w324, new element=w323) -> (w322:string[])  [unwired: 1 in]
                  n196 = case shown="\"结束\"" w320 {
                    selector: w320 -> [w349 w352 w355]
                    tunnel: [w349 w351 w354] -> w319
                    frame Default {
                    }
                    frame "初始化" {
                      n197 = Concatenate Strings("-->>" ("字符串"), w352) -> (w351:string)
                    }
                    frame "结束" {
                      n198 = Concatenate Strings("-->>" ("字符串"), w355) -> (w354:string)
                    }
                  }
                  n199 = global read "VAR总磷全局变量.vi" "状态告警区"() -> (w317:T4)
                  n200 = Unbundle By Name(w317) -> ("工作状态"=w316:T9)
                  n201 = global read "VAR总磷全局变量.vi" "状态告警区"() -> (w339:T4)
                  n202 = case shown="\"水样测试\"" w316 {
                    tunnel: [_ "【水样测试】" ("字符串") "【标样核查】" ("字符串") "【零点核查】" ("字符串") "【跨度核查】" ("字符串") "【空白测试】" ("字符串") "【平行样测试】" ("字符串") "【加标回收】" ("字符串") "【空白校准】" ("字符串") "【标样校准】" ("字符串")] -> w315
                    frame "空闲", Default {
                    }
                    frame "水样测试" {
                    }
                    frame "标样核查" {
                    }
                    frame "零点核查" {
                    }
                    frame "跨度核查" {
                    }
                    frame "空白测试" {
                    }
                    frame "平行样测试" {
                    }
                    frame "加标回收" {
                    }
                    frame "空白校准" {
                    }
                    frame "标样校准" {
                    }
                  }
                  n203 = Unbundle By Name(w339) -> ("id"=w338:u16)
                  n204 = global read "VAR总磷全局变量.vi" "状态告警区"() -> (w334:T4)
                  n205 = case shown="1, 131" w338 {
                    tunnel: [_ "总磷" ("table输入") "氨氮" ("table输入") "总氮" ("table输入")] -> w336
                    frame Default {
                    }
                    frame 1, 131 {
                    }
                    frame 3, 92 {
                    }
                    frame 2, 76 {
                    }
                  }
                  n206 = Unbundle By Name(w334) -> ("F0"=w331:sgl, "F1"=w330:sgl, "F2"=w329:sgl, "F3"=w328:sgl, "id"=w327:u16, "flowid"=w326:u16, "量程"=w325:u16)
                  n207 = Concatenate Strings(w315, w319) -> (w318:string)
                  n208 = Format Into String(format string="F0=%#f,F1=%#f,F2=%#f,F3=%#f,Flow=%d-%-d-%-d" ("格式字符串"), w331, w330, w329, w328, w327, w326, w325) -> (resulting string=w332:string)  [unwired: 2 in, 1 out]
                  n209 = Get Date/Time In Seconds() -> (seconds since 1Jan1904=w335:timestamp)
                  n210 = Bundle By Name(cluster=T16 {"时间标识"=timestamp(0 s since 1904-01-01), "设备"="", "日志信息"="", "流程参数"=""} ("data in"), "时间标识"=w335, "设备"=w336, "日志信息"=w318, "流程参数"=w332) -> (w337:T16)
                  n211 = call "总磷操作日志.vi"("data in"=w337) -> ()  [unwired: 11 in]
                }
              }
            }
            n212 = local write "数组"(w300) -> ()
          }
        }
      }
    }
    n213 = call <vilib>:"Boolean Crossing PtByPt.vi"("input"=w242) -> ("crossing"=w206:bool)  [unwired: 2 in]
    n214 = Bundle By Name(cluster=T15 {"启动模式"=enum."跨度核查", "启动参数"=1, "量程"=enum."低量程"} ("参数簇"), "启动参数"=w237, "启动模式"=w239, "量程"=w238) -> (w231:T15)
    n215 = First Call?() -> (First Call?: T/F=w243:bool)
    n216 = Or(x=w206, y=w243) -> (x .or. y?=w241:bool)
    n217 = while {
      tunnel: w241 -> [w444]
      tunnel: w231 -> [w443]
      shift-right: [w438] -> _
      shift-left: _ -> [w440]
      shift-right: [w439] -> _
      shift-left: _ -> [w441]
      stop <- TRUE stop-if-true
      n218 = case shown="真" w444 {
        tunnel: [w446 w454] -> w439
        tunnel: [w445 w453] -> w438
        tunnel: w443 -> [_ w448]
        tunnel: w441 -> [w446 _]
        tunnel: w440 -> [w445 _]
        frame False {
        }
        frame True {
          n219 = call "斯坦道XML解析.vi"("添加的路径"="流程路径", "参数簇"=w448) -> ("步骤时间"=w449:string[], "步骤名"=w451:string[])  [unwired: 8 in]
          n220 = for {
            tunnel: w451 -> [_] mode=indexing
            tunnel: [w455] -> w452 mode=indexing
            i -> [w455]
          }
          n221 = Build Array(w451, w449) -> (w450:string[][])
          n222 = Transpose 2D Array(2D array=w450) -> (transposed array=w453:string[][])
          n223 = Number To Decimal String(number=w452) -> (decimal integer string=w454:string[])  [unwired: 1 in]
        }
      }
      n224 = property on="多列列表框" class="MCListbox (严格)"("ItemNames"=w438, "RowHdrs[]"=w439) -> ()  [unwired: 2 in, 2 out]
    }
    n225 = case shown="1, 默认" w225 {
      selector: w225 -> [_ w385]
      tunnel: w228 -> [_ w386]
      tunnel: w227 -> [_ w384]
      frame 0 {
      }
      frame 1, Default {
        n226 = case shown="真" w384 {
          tunnel: w386 -> [_ w393]
          tunnel: w385 -> [_ w387]
          frame False {
          }
          frame True {
            n227 = case shown="默认" w387 {
              selector: w387 -> [w395 _ _ _ _ _ _ _ _ _ _ _ _ _ _ _ _ _ _ _ _ _ _ _ _ _ _ _ _ _ _ _ _ _ _ _ _ _]
              tunnel: [w394 "无告警" "缺试剂告警" "缺水样告警" "缺蒸馏水告警" "缺标液告警" "仪表漏液告警" "标定异常告警" "超量程告警" "加热异常" "低试剂预警" "超上限告警" "超下限告警" "仪表内部其他异常" "滴定异常告警" "电极异常告警" "量程切换告警" "参数设置告警" "PH电极电位异常" "电导率电极异常" "浊度光度异常" "溶解氧电极异常" "溶解氧光强异常" "温度异常告警" "PH异常告警" "溶解氧异常告警" "电导率异常告警" "浊度异常告警" "叶绿素异常告警" "藻密度异常告警" "蓝绿藻异常告警" "ORP异常告警" "氨氮异常告警" "清洁刷异常告警" "SD卡异常告警" "蓝牙异常告警" "WiFi异常告警" "流程异常告警"] -> w388
              frame Default {
                n228 = Format Into String(format string="%d" ("格式字符串"), initial string="内部告警-" ("工作状态"), w395) -> (resulting string=w394:string)  [unwired: 1 in, 1 out]
              }
              frame 0 {
              }
              frame 1 {
              }
              frame 2 {
              }
              frame 3 {
              }
              frame 4 {
              }
              frame 5 {
              }
              frame 6 {
              }
              frame 7 {
              }
              frame 8 {
              }
              frame 9 {
              }
              frame 10 {
              }
              frame 11 {
              }
              frame 12 {
              }
              frame 13 {
              }
              frame 14 {
              }
              frame 15 {
              }
              frame 16 {
              }
              frame 17 {
              }
              frame 18 {
              }
              frame 19 {
              }
              frame 20 {
              }
              frame 21 {
              }
              frame 22 {
              }
              frame 23 {
              }
              frame 24 {
              }
              frame 25 {
              }
              frame 26 {
              }
              frame 27 {
              }
              frame 28 {
              }
              frame 29 {
              }
              frame 30 {
              }
              frame 31 {
              }
              frame 32 {
              }
              frame 33 {
              }
              frame 34 {
              }
              frame 35 {
              }
              frame 36 {
              }
            }
            n229 = case shown="2, 76, 默认" w393 {
              tunnel: ["总磷" ("table输入") "氨氮" ("table输入") "总氮" ("table输入")] -> w389
              frame 1, 131 {
              }
              frame 3, 92 {
              }
              frame 2, 76, Default {
              }
            }
            n230 = Get Date/Time In Seconds() -> (seconds since 1Jan1904=w390:timestamp)
            n231 = Bundle By Name(cluster=T17 {"时间标识"=timestamp(0 s since 1904-01-01), "设备"="", "日志信息"=""} ("data in"), "时间标识"=w390, "设备"=w389, "日志信息"=w388) -> (w391:T17)
            n232 = call "总磷报警信息.vi"("data in"=w391) -> ()  [unwired: 10 in, 1 out]
          }
        }
      }
    }
  }
  n233 = Bundle("参数下拉列表"=w4, "测量模式下拉列表"=w3, "量程下拉列表"=w2) -> (w5:T19)  [unwired: 1 in]
  n234 = Obtain Notifier(name (unnamed)="TP" ("名称（未命名）"), notification data type=FALSE) -> (notifier out=w8:refnum<notifier>)  [unwired: 2 in, 2 out]
  n235 = property on="曲线模型" class="曲线模型 (严格)"("属性"=w5) -> (error out=w11:errorcluster)  [unwired: 2 in, 1 out]
  n236 = Cancel Notification(0:w8) -> (8:w7:refnum<notifier>)  [unwired: 1 in, 2 out]
  n237 = control-ref of="测量模式下拉列表"() -> (w17:refnum<vi>)
  n238 = control-ref of="量程参数读取"() -> (w6:refnum<vi>)
  n239 = control-ref of="参数下拉列表"() -> (w18:refnum<vi>)
  n240 = control-ref of="量程下拉列表"() -> (w19:refnum<vi>)
  n241 = control-ref of="公式"() -> (w16:refnum<vi>)
  n242 = Obtain Queue(name (unnamed)="TP" ("名称（未命名）"), element data type=cluster{"命令":string, "data":variant} {"命令"="", "data"=variant}) -> (queue out=w20:refnum<queue>, error out=w21:errorcluster)  [unwired: 3 in, 1 out]
  n243 = while {
    tunnel: w20 -> [w472]
    tunnel: w21 -> [_]
    stop <- FALSE stop-if-true
    n244 = Get Queue Status(queue=w472) -> (queue out=w468:refnum<queue>, # elements in queue=w467:i32)  [unwired: 2 in, 6 out]
    n245 = Wait (ms)(milliseconds to wait=u32 1000 ("等待时间（毫秒）")) -> ()  [unwired: 1 out]
    n246 = case shown="0" w467 {
      tunnel: w468 -> [_ w488]
      frame Default {
      }
      frame 0 {
        w483 = u16 1 items=["总磷"=1, "氨氮"=3] ("站号")
        # "试剂填充 172 \n管路清洗108\n氨氮92\n总磷131\n总磷海水147\n总氮76\n总氮海水92"
        n247 = Bundle By Name(cluster=cluster{"命令":string, "data":variant} {"命令"="", "data"=variant} ("元素"), "命令"="读状态告警区", "data"=w483) -> (w490:cluster{"命令":string, "data":variant})
        n248 = Bundle By Name(cluster=cluster{"命令":string, "data":variant} {"命令"="", "data"=variant} ("元素"), "命令"="读测量数据区", "data"=w483) -> (w486:cluster{"命令":string, "data":variant})
        n249 = global read "VAR总磷全局变量.vi" "状态告警区"() -> (w475:T4)
        n250 = Unbundle By Name(w475) -> ("系统时间"=w482:timestamp)
        n251 = Enqueue Element(queue=w488, element=w490) -> (queue out=w484:refnum<queue>)  [unwired: 2 in, 2 out]
        n252 = Get Date/Time In Seconds() -> (seconds since 1Jan1904=w481:timestamp)
        n253 = Subtract(x=w481, y=w482) -> (x-y=w480:dbl)
        n254 = Absolute Value(x=w480) -> (abs(x)=w479:dbl)
        n255 = Enqueue Element(queue=w484, element=w486) -> (queue out=w476:refnum<queue>)  [unwired: 2 in, 2 out]
        n256 = Greater Or Equal?(x=w479, y=120.0) -> (x >= y?=w477:bool)
        n257 = case shown="真" w477 {
          tunnel: w476 -> [_ w493]
          frame False {
          }
          frame True {
            n258 = call "总磷启动命令.vi"("参数"=T20 {"站号"=3, "量程切换"=enum."AUTO", "控制命令"=enum."校时", "模式设置"=enum."待机", "测量间隔"=0}) -> ("启动命令"=w492:cluster{"命令":string, "data":variant})  [unwired: 10 in]
            n259 = Enqueue Element(queue=w493, element=w492) -> ()  [unwired: 2 in, 3 out]
          }
        }
      }
    }
    n260 = global read "总磷断电保存全局变量.vi" "流程路径"() -> (w471:path)
    n261 = global read "总磷断电保存全局变量.vi" "MB通信方式选择"() -> (w469:enum16{"串口", "TCP"})
    n262 = local write "流程路径"(w471) -> ()
    n263 = case shown="\"TCP\"" w469 {
      tunnel: [w495 w496] -> w470
      frame "串口", Default {
        n264 = global read "总磷断电保存全局变量.vi" "VISA Resource"() -> (w495:refnum<visa-resource-name>)
      }
      frame "TCP" {
        n265 = global read "总磷断电保存全局变量.vi" "IP"() -> (w496:string)
      }
    }
    "字符串" <- w470
  }
  n266 = while {
    tunnel: w20 -> [w503]
    tunnel: w19 -> [w502]
    tunnel: w18 -> [w501]
    tunnel: w17 -> [w500]
    tunnel: w16 -> [w499]
    tunnel: w6 -> [w498]
    tunnel: w11 -> [_]
    tunnel: w7 -> [w497]
    stop <- FALSE stop-if-true
    n267 = event shown="[1] \"权限锁\": 鼠标按下" {
      selector: _ -> [_ _ _ _ _ _ _ _ _ _ _ _ _ _ _ _ _ _ _ _ _ _ _]
      dyn-events: _ -> [_ _ _ _ _ _ _ _ _ _ _ _ _ _ _ _ _ _ _ _ _ _ _]
      timeout: _ -> [_ _ _ _ _ _ _ _ _ _ _ _ _ _ _ _ _ _ _ _ _ _ _]
      tunnel: w503 -> [_ _ _ _ w523 w551 _ _ _ _ _ _ w653 _ w678 w685 _ _ _ _ _ _ _]
      tunnel: w502 -> [_ _ _ _ _ _ _ _ _ _ _ _ _ _ _ _ _ _ _ w701 _ _ _]
      tunnel: w501 -> [_ _ _ _ _ _ _ _ _ _ _ _ _ _ _ _ _ _ _ w699 _ w717 w724]
      tunnel: w500 -> [_ _ _ _ _ _ _ _ _ _ _ _ _ _ _ _ _ _ _ w700 _ _ _]
      tunnel: w499 -> [_ _ _ _ _ _ _ _ _ _ _ _ _ _ _ _ _ _ _ w695 _ _ _]
      tunnel: w498 -> [_ _ _ _ _ _ _ _ _ _ _ _ _ _ _ _ _ _ _ _ _ w715 _]
      tunnel: w497 -> [_ _ _ _ _ _ _ _ _ _ _ _ _ _ _ w680 _ _ _ _ _ _ _]
      tunnel: [_ _ _ w509 _ _ _ _ _ _ _ _ _ _ _ _ _ _ _ _ _ _ _] -> _
      event Timeout {
        n268 = event-data() -> ()  [unwired: 1 in, 3 out]
      }
      event "权限锁": Mouse Down {
        n269 = event-data() -> ("CtlRef"=w506:refnum<vi>)  [unwired: 1 in, 5 out]
        n270 = property class="Bool (严格)"(reference=w506) -> ("Value"=w505:bool)  [unwired: 1 in, 2 out]
        n271 = case shown="真" w505 {
          frame False {
            n272 = call "密码键盘.vi"() -> ("NewNumber"=→"输入密码":dbl)  [unwired: 1 in]
          }
          frame True {
            n273 = local write "输入密码"(u32 0 ("输入密码")) -> ()
          }
        }
      }
      event "流程固件": Value Change {
        n274 = event-data() -> ()  [unwired: 1 in, 6 out]
        n275 = call "流程固件设置对话框.vi"() -> ()  [unwired: 12 in]
      }
      event "测量模式下拉列表", "量程下拉列表", "参数下拉列表": Value Change {
        n276 = event-data() -> ()  [unwired: 1 in, 6 out]
        n277 = local read "测量模式下拉列表"() -> (w512:enum16{"水样测量", "零点核查", "跨度核查", "标样核查", "加标回收"})
        n278 = local read "参数下拉列表"() -> (w511:enum16{"总磷", "总氮"})
        n279 = local read "量程下拉列表"() -> (w513:enum16{"低量程", "高量程"})
        n280 = Bundle("参数下拉列表"=w511, "测量模式下拉列表"=w512, "量程下拉列表"=w513) -> (w510:T19)  [unwired: 1 in]
        n281 = property on="曲线模型" class="曲线模型 (严格)"("属性"=w510) -> (error out=w509:errorcluster)  [unwired: 2 in, 1 out]
      }
      event "串口设置": Value Change {
        n282 = event-data() -> ()  [unwired: 1 in, 6 out]
        n283 = global read "总磷断电保存全局变量.vi" "MB通信方式选择"() -> (w514:enum16{"串口", "TCP"})
        n284 = global read "总磷断电保存全局变量.vi" "VISA Resource"() -> (w520:refnum<visa-resource-name>)
        n285 = global read "总磷断电保存全局变量.vi" "PORT"() -> (w518:string)
        n286 = global read "总磷断电保存全局变量.vi" "IP"() -> (w519:string)
        n287 = call "串口配置.vi"("PORT"=w518, "IP"=w519, "MB通信方式选择"=w514, "请选择串口:"=w520) -> ("PORT 2"=w516:string, "IP 2"=w517:string, "确认 2"=w521:bool, "VISA资源名称 2"=w522:refnum<visa-resource-name>, "MB通信方式选择 2"=w515:enum16{"串口", "TCP"})  [unwired: 3 in]
        n288 = case shown="真" w521 {
          tunnel: w522 -> [_ w528]
          tunnel: w523 -> [_ w527]
          tunnel: w517 -> [_ w526]
          tunnel: w516 -> [_ w525]
          tunnel: w515 -> [_ w524]
          frame False {
          }
          frame True {
            n289 = flat-sequence {
              tunnel: w528 -> [w533]
              tunnel: w527 -> [w534]
              tunnel: w526 -> [w532]
              tunnel: w525 -> [w531]
              tunnel: w524 -> [w530]
              frame #0 {
                n290 = global write "总磷断电保存全局变量.vi" "IP"(w532) -> ()
                n291 = global write "总磷断电保存全局变量.vi" "PORT"(w531) -> ()
                n292 = global write "总磷断电保存全局变量.vi" "VISA Resource"(w533) -> ()
                n293 = global write "总磷断电保存全局变量.vi" "MB通信方式选择"(w530) -> ()
                n294 = Flush Queue(queue=w534) -> (queue out=w529:refnum<queue>)  [unwired: 1 in, 2 out]
                n295 = Enqueue Element(queue=w529, element=cluster{"命令":string, "data":variant} {"命令"="启用模块", "data"=variant} ("元素")) -> ()  [unwired: 2 in, 3 out]
              }
              frame #1 {
                n296 = call <vilib>:"Application Directory.vi"() -> ("Application Directory"=w549:path)
                n297 = Build Path(base path=w549, name or relative path="data\\sys.ini" ("名称或相对路径")) -> (appended path=w547:path)
                n298 = call <vilib>:"Open Config Data.vi"("configuration file path"=w547) -> ("error out"=w543:errorcluster, "refnum"=w546:T13)  [unwired: 8 in, 1 out]
                n299 = vi-ref "总磷断电保存全局变量.vi"() -> (w545:refnum<vi>)
                n300 = call <userlib>:"Write Panel to INI__ogtk.vi"("error in (no error)"=w543, "VI ref"=w545, "refnum"=w546) -> ("error out"=w542:errorcluster, "refnum out"=w544:T13)  [unwired: 7 in]
                n301 = call <vilib>:"Close Config Data.vi"("error in (no error)"=w542, "refnum"=w544) -> ("error out"=w537:errorcluster, "file path"=w536:path)  [unwired: 8 in]
                n302 = Open/Create/Replace File(file path (use dialog)=w536, error in=w537) -> (refnum out=w540:refnum<file>, error out=w541:errorcluster)  [unwired: 4 in, 1 out]
                n303 = Flush File(refnum=w540, error in=w541) -> (refnum out=w539:refnum<file>, error out=w538:errorcluster)
                n304 = Close File(refnum=w539, error in=w538) -> ()  [unwired: 2 out]
              }
            }
          }
        }
      }
      event "模块启用": Value Change {
        n305 = event-data() -> ("OldVal"=w552:bool)  [unwired: 1 in, 5 out]
        n306 = Flush Queue(queue=w551) -> (queue out=w550:refnum<queue>)  [unwired: 1 in, 2 out]
        n307 = case shown="假" w552 {
          tunnel: w550 -> [w553 w555]
          frame False {
            n308 = Enqueue Element(queue=w553, element=cluster{"命令":string, "data":variant} {"命令"="停用模块", "data"=variant} ("元素")) -> ()  [unwired: 2 in, 3 out]
          }
          frame True {
            n309 = Enqueue Element(queue=w555, element=cluster{"命令":string, "data":variant} {"命令"="启用模块", "data"=variant} ("元素")) -> ()  [unwired: 2 in, 3 out]
          }
        }
      }
      event "流程路径": Value Change {
        n310 = event-data() -> ()  [unwired: 1 in, 6 out]
        n311 = flat-sequence {
          frame #0 {
            n312 = local read "流程路径"() -> (w557:path)
            n313 = global write "总磷断电保存全局变量.vi" "流程路径"(w557) -> ()
          }
          frame #1 {
            n314 = call <vilib>:"Application Directory.vi"() -> ("Application Directory"=w571:path)
            n315 = Build Path(base path=w571, name or relative path="data\\sys.ini" ("名称或相对路径")) -> (appended path=w569:path)
            n316 = call <vilib>:"Open Config Data.vi"("configuration file path"=w569) -> ("error out"=w565:errorcluster, "refnum"=w568:T13)  [unwired: 8 in, 1 out]
            n317 = vi-ref "总磷断电保存全局变量.vi"() -> (w567:refnum<vi>)
            n318 = call <userlib>:"Write Panel to INI__ogtk.vi"("error in (no error)"=w565, "VI ref"=w567, "refnum"=w568) -> ("error out"=w564:errorcluster, "refnum out"=w566:T13)  [unwired: 7 in]
            n319 = call <vilib>:"Close Config Data.vi"("error in (no error)"=w564, "refnum"=w566) -> ("error out"=w559:errorcluster, "file path"=w558:path)  [unwired: 8 in]
            n320 = Open/Create/Replace File(file path (use dialog)=w558, error in=w559) -> (refnum out=w562:refnum<file>, error out=w563:errorcluster)  [unwired: 4 in, 1 out]
            n321 = Flush File(refnum=w562, error in=w563) -> (refnum out=w561:refnum<file>, error out=w560:errorcluster)
            n322 = Close File(refnum=w561, error in=w560) -> ()  [unwired: 2 out]
          }
        }
      }
      event "公式一键写入": Value Change {
        n323 = event-data() -> ()  [unwired: 1 in, 6 out]
        n324 = local read "公式"() -> (w572:cluster{"X^2":dbl, "X":dbl, "b":dbl})
        n325 = call "公式复合写入.vi"("公式"=w572) -> ()  [unwired: 11 in]
      }
      event "曲线模型": Value Change {
        n326 = event-data() -> ()  [unwired: 1 in, 6 out]
        n327 = local write "公式"("曲线模型") -> ()
      }
      event "质控参数设置": Value Change {
        n328 = event-data() -> ()  [unwired: 1 in, 6 out]
        n329 = global read "总磷断电保存全局变量.vi" "质控参数设置"() -> (w574:T21)
        n330 = call "总磷质控参数设置.vi"("质控参数设置"=w574) -> ("输出簇"=w575:T22)  [unwired: 10 in]
        n331 = Unbundle By Name(w575) -> ("确定"=w576:bool)
        n332 = case shown="真" w576 {
          tunnel: w575 -> [_ w578]
          tunnel: w574 -> [_ w577]
          frame False {
          }
          frame True {
            n333 = flat-sequence {
              tunnel: w578 -> [w585]
              tunnel: w577 -> [w584]
              frame #0 {
                n334 = Unbundle By Name(w585) -> ("总磷跨度值"=w583:dbl, "总磷零点标准液浓度"=w582:dbl, "总磷跨度标准液浓度"=w581:dbl, "总磷标准液标准浓度"=w580:dbl)
                n335 = Bundle By Name(cluster=w584, "总磷跨度值"=w583, "总磷零点标准液浓度"=w582, "总磷跨度标准液浓度"=w581, "总磷标准液标准浓度"=w580) -> (w579:T21)
                n336 = global write "总磷断电保存全局变量.vi" "质控参数设置"(w579) -> ()
              }
              frame #1 {
                n337 = call <vilib>:"Application Directory.vi"() -> ("Application Directory"=w599:path)
                n338 = Build Path(base path=w599, name or relative path="data\\sys.ini" ("名称或相对路径")) -> (appended path=w597:path)
                n339 = call <vilib>:"Open Config Data.vi"("configuration file path"=w597) -> ("error out"=w593:errorcluster, "refnum"=w596:T13)  [unwired: 8 in, 1 out]
                n340 = vi-ref "总磷断电保存全局变量.vi"() -> (w595:refnum<vi>)
                n341 = call <userlib>:"Write Panel to INI__ogtk.vi"("error in (no error)"=w593, "VI ref"=w595, "refnum"=w596) -> ("error out"=w592:errorcluster, "refnum out"=w594:T13)  [unwired: 7 in]
                n342 = call <vilib>:"Close Config Data.vi"("error in (no error)"=w592, "refnum"=w594) -> ("error out"=w587:errorcluster, "file path"=w586:path)  [unwired: 8 in]
                n343 = Open/Create/Replace File(file path (use dialog)=w586, error in=w587) -> (refnum out=w590:refnum<file>, error out=w591:errorcluster)  [unwired: 4 in, 1 out]
                n344 = Flush File(refnum=w590, error in=w591) -> (refnum out=w589:refnum<file>, error out=w588:errorcluster)
                n345 = Close File(refnum=w589, error in=w588) -> ()  [unwired: 2 out]
              }
            }
          }
        }
      }
      event "仪器参数设置": Value Change {
        n346 = event-data() -> ()  [unwired: 1 in, 6 out]
        n347 = global read "总磷断电保存全局变量.vi" "总磷仪器参数"() -> (w601:T23)
        n348 = call "仪器参数设置.vi"("仪器参数设置"=w601) -> ("仪器参数设置输出"=w600:T24)  [unwired: 10 in]
        n349 = Unbundle By Name(w600) -> ("确定"=w602:bool)
        n350 = case shown="真" w602 {
          tunnel: w600 -> [_ w604]
          tunnel: w601 -> [_ w603]
          frame False {
          }
          frame True {
            n351 = flat-sequence {
              tunnel: w604 -> [w621]
              tunnel: w603 -> [w620]
              frame #0 {
                n352 = Unbundle By Name(w621) -> ("测量量程"=w619:dbl, "测量精度"=w618:dbl, "测量间隔"=w617:dbl, "消解温度"=w616:dbl, "消解时长"=w614:dbl, "空白校准时间"=w613:timestamp, "曲线截距"=w612:dbl, "曲线斜率"=w611:dbl, "测量检出限"=w610:dbl, "测量信号值"=w609:dbl, "线性相关系数"=w608:dbl, "二次多项式系数"=w607:dbl, "标样校准时间"=w606:timestamp, "单位"=w605:u16)
                n353 = Bundle By Name(cluster=w620, "测量量程"=w619, "测量精度"=w618, "测量间隔"=w617, "消解温度"=w616, "消解时长"=w614, "空白校准时间"=w613, "曲线截距"=w612, "曲线斜率"=w611, "测量检出限"=w610, "测量信号值"=w609, "线性相关系数"=w608, "二次多项式系数"=w607, "标样校准时间"=w606, "单位"=w605) -> (w615:T23)
                n354 = global write "总磷断电保存全局变量.vi" "总磷仪器参数"(w615) -> ()
              }
              frame #1 {
                n355 = call <vilib>:"Application Directory.vi"() -> ("Application Directory"=w635:path)
                n356 = Build Path(base path=w635, name or relative path="data\\sys.ini" ("名称或相对路径")) -> (appended path=w633:path)
                n357 = call <vilib>:"Open Config Data.vi"("configuration file path"=w633) -> ("error out"=w629:errorcluster, "refnum"=w632:T13)  [unwired: 8 in, 1 out]
                n358 = vi-ref "总磷断电保存全局变量.vi"() -> (w631:refnum<vi>)
                n359 = call <userlib>:"Write Panel to INI__ogtk.vi"("error in (no error)"=w629, "VI ref"=w631, "refnum"=w632) -> ("error out"=w628:errorcluster, "refnum out"=w630:T13)  [unwired: 7 in]
                n360 = call <vilib>:"Close Config Data.vi"("error in (no error)"=w628, "refnum"=w630) -> ("error out"=w623:errorcluster, "file path"=w622:path)  [unwired: 8 in]
                n361 = Open/Create/Replace File(file path (use dialog)=w622, error in=w623) -> (refnum out=w626:refnum<file>, error out=w627:errorcluster)  [unwired: 4 in, 1 out]
                n362 = Flush File(refnum=w626, error in=w627) -> (refnum out=w625:refnum<file>, error out=w624:errorcluster)
                n363 = Close File(refnum=w625, error in=w624) -> ()  [unwired: 2 out]
              }
            }
          }
        }
      }
      event "总磷自动测试量程配置": Value Change {
        n364 = event-data() -> ()  [unwired: 1 in, 6 out]
        n365 = flat-sequence {
          frame #0 {
            n366 = global write "总磷断电保存全局变量.vi" "总磷自动测试量程配置"("总磷自动测试量程配置") -> ()
          }
          frame #1 {
            n367 = call <vilib>:"Application Directory.vi"() -> ("Application Directory"=w650:path)
            n368 = Build Path(base path=w650, name or relative path="data\\sys.ini" ("名称或相对路径")) -> (appended path=w648:path)
            n369 = call <vilib>:"Open Config Data.vi"("configuration file path"=w648) -> ("error out"=w644:errorcluster, "refnum"=w647:T13)  [unwired: 8 in, 1 out]
            n370 = vi-ref "总磷断电保存全局变量.vi"() -> (w646:refnum<vi>)
            n371 = call <userlib>:"Write Panel to INI__ogtk.vi"("error in (no error)"=w644, "VI ref"=w646, "refnum"=w647) -> ("error out"=w643:errorcluster, "refnum out"=w645:T13)  [unwired: 7 in]
            n372 = call <vilib>:"Close Config Data.vi"("error in (no error)"=w643, "refnum"=w645) -> ("error out"=w638:errorcluster, "file path"=w637:path)  [unwired: 8 in]
            n373 = Open/Create/Replace File(file path (use dialog)=w637, error in=w638) -> (refnum out=w641:refnum<file>, error out=w642:errorcluster)  [unwired: 4 in, 1 out]
            n374 = Flush File(refnum=w641, error in=w642) -> (refnum out=w640:refnum<file>, error out=w639:errorcluster)
            n375 = Close File(refnum=w640, error in=w639) -> ()  [unwired: 2 out]
          }
        }
      }
      event "手动启动": Value Change {
        n376 = event-data() -> ()  [unwired: 1 in, 6 out]
        n377 = call "总磷启动参数对话框.vi"() -> ("确认"=w651:bool, "元素"=w652:cluster{"命令":string, "data":variant})  [unwired: 10 in]
        n378 = case shown="真" w651 {
          tunnel: w653 -> [_ w655]
          tunnel: w652 -> [_ w654]
          frame False {
          }
          frame True {
            n379 = Enqueue Element(queue=w655, element=w654) -> ()  [unwired: 2 in, 3 out]
          }
        }
      }
      event "定时启动": Mouse Down {
        n380 = event-data() -> ()  [unwired: 1 in, 6 out]
        n381 = flat-sequence {
          frame #0 {
            n382 = global read "总磷断电保存全局变量.vi" "定时控制"() -> (w657:T6)
            n383 = call "总磷周期设置.vi"("定时控制输入"=w657) -> ("定时控制输出"=w656:T25)  [unwired: 10 in]
            n384 = global write "总磷断电保存全局变量.vi" "定时控制"(w656) -> ()
          }
          frame #1 {
            n385 = call <vilib>:"Application Directory.vi"() -> ("Application Directory"=w671:path)
            n386 = Build Path(base path=w671, name or relative path="data\\sys.ini" ("名称或相对路径")) -> (appended path=w669:path)
            n387 = call <vilib>:"Open Config Data.vi"("configuration file path"=w669) -> ("error out"=w665:errorcluster, "refnum"=w668:T13)  [unwired: 8 in, 1 out]
            n388 = vi-ref "总磷断电保存全局变量.vi"() -> (w667:refnum<vi>)
            n389 = call <userlib>:"Write Panel to INI__ogtk.vi"("error in (no error)"=w665, "VI ref"=w667, "refnum"=w668) -> ("error out"=w664:errorcluster, "refnum out"=w666:T13)  [unwired: 7 in]
            n390 = call <vilib>:"Close Config Data.vi"("error in (no error)"=w664, "refnum"=w666) -> ("error out"=w659:errorcluster, "file path"=w658:path)  [unwired: 8 in]
            n391 = Open/Create/Replace File(file path (use dialog)=w658, error in=w659) -> (refnum out=w662:refnum<file>, error out=w663:errorcluster)  [unwired: 4 in, 1 out]
            n392 = Flush File(refnum=w662, error in=w663) -> (refnum out=w661:refnum<file>, error out=w660:errorcluster)
            n393 = Close File(refnum=w661, error in=w660) -> ()  [unwired: 2 out]
          }
        }
      }
      event "单步测试": Value Change {
        w673 = u16 1 items=["总磷"=1, "氨氮"=3] ("站号")
        n394 = event-data() -> ()  [unwired: 1 in, 6 out]
        n395 = Bundle("站号"=w673, "总磷氨氮调试"="总磷氨氮调试") -> (w672:cluster{"站号":u16, "总磷氨氮调试":u16[]})  [unwired: 1 in]
        n396 = Bundle By Name(cluster=cluster{"命令":string, "data":variant} {"命令"="", "data"=variant} ("元素"), "命令"="debug", "data"=w672) -> (w675:cluster{"命令":string, "data":variant})
        n397 = Enqueue Element(queue=w678, element=w675) -> ()  [unwired: 2 in, 3 out]
      }
      event "停止": Value Change {
        n398 = event-data() -> ()  [unwired: 1 in, 6 out]
        n399 = Enqueue Element(queue=w685, element=cluster{"命令":string, "data":variant} {"命令"="启动", "data"=variant(cluster{"站号":u16, "控制命令输出":u16[]} {"站号"=1, "控制命令输出"=[2816]})} ("元素")) -> (queue out=w682:refnum<queue>)  [unwired: 2 in, 2 out]
        n400 = Cancel Notification(0:w680) -> (8:w681:refnum<notifier>)  [unwired: 1 in, 2 out]
        n401 = Send Notification(notification=TRUE ("通知"), notifier=w681) -> ()  [unwired: 1 in, 2 out]
        n402 = Enqueue Element(queue=w682, element=cluster{"命令":string, "data":variant} {"命令"="启动", "data"=variant(cluster{"站号":u16, "控制命令输出":u16[]} {"站号"=2, "控制命令输出"=[2816]})} ("元素")) -> ()  [unwired: 2 in, 3 out]
      }
      event "设置": Value Change {
        n403 = event-data() -> ()  [unwired: 1 in, 6 out]
        n404 = property on="窗格" class="Pane"("Origin"=T11 {"Horizontal"=0, "Vertical"=628} ("原点")) -> ()  [unwired: 2 in, 2 out]
      }
      event "返回": Value Change {
        n405 = event-data() -> ()  [unwired: 1 in, 6 out]
        n406 = property on="窗格" class="Pane"("Origin"=T11 {"Horizontal"=0, "Vertical"=0} ("原点")) -> ()  [unwired: 2 in, 2 out]
      }
      event "公式.X^2", "公式.X", "公式.b": Mouse Down {
        n407 = event-data() -> ("CtlRef"=w691:refnum<vi>)  [unwired: 1 in, 5 out]
        n408 = property class="DigNum (严格)"(reference=w691) -> (reference out=w689:refnum<vi>, "Value"=w690:dbl)  [unwired: 1 in, 1 out]
        n409 = call "数字键盘.vi"("OldNumber"=w690) -> ("NewNumber"=w688:dbl)
        n410 = property class="DigNum (严格)"(reference=w689, "Val(Sgnl)"=w688) -> ()  [unwired: 1 in, 2 out]
      }
      event "读公式": Value Change {
        n411 = event-data() -> ()  [unwired: 1 in, 6 out]
        n412 = property class="Enum (严格)"(reference=w699) -> ("Value"=w698:enum16{"总磷", "总氮"})  [unwired: 1 in, 2 out]
        n413 = property class="Enum (严格)"(reference=w700) -> ("Value"=w697:enum16{"水样测量", "零点核查", "跨度核查", "标样核查", "加标回收"})  [unwired: 1 in, 2 out]
        n414 = property class="Enum (严格)"(reference=w701) -> ("Value"=w696:enum16{"低量程", "高量程"})  [unwired: 1 in, 2 out]
        n415 = call "总磷总氮公式读取.vi"("量程"=w696, "测量模式"=w697, "测量参数"=w698) -> ("error out"=w693:errorcluster, "公式"=w694:cluster{"X^2":dbl, "X":dbl, "b":dbl})  [unwired: 7 in]
        n416 = property class="Clust (严格)"(reference=w695, "Value"=w694) -> ()  [unwired: 1 in, 2 out]
        n417 = case shown="错误" w693 {
          tunnel: ["读取成功" ("消息") "读取失败" ("消息")] -> w692
          frame No Error {
          }
          frame Error {
          }
        }
        n418 = One Button Dialog(message=w692) -> ()  [unwired: 1 in, 1 out]
      }
      event "写公式": Value Change {
        n419 = event-data() -> ()  [unwired: 1 in, 6 out]
        n420 = call "总磷总氮公式写入.vi"("公式"="公式", "量程"="量程下拉列表", "测量模式"="测量模式下拉列表", "测量参数"="参数下拉列表") -> ("error out"=w706:errorcluster)  [unwired: 7 in]
        n421 = case shown="无错误" w706 {
          tunnel: ["写入成功" ("消息") "写入失败" ("消息")] -> w707
          frame No Error {
          }
          frame Error {
          }
        }
        n422 = One Button Dialog(message=w707) -> ()  [unwired: 1 in, 1 out]
      }
      event "量程切换阈值读取": Value Change {
        n423 = event-data() -> ()  [unwired: 1 in, 6 out]
        n424 = property class="Enum (严格)"(reference=w717) -> ("Value"=w716:enum16{"总磷", "总氮"})  [unwired: 1 in, 2 out]
        n425 = call "总磷总氮量程读取.vi"("测量参数"=w716) -> ("error out"=w712:errorcluster, "量程参数读取"=w714:T26)  [unwired: 9 in]
        n426 = property class="Clust (严格)"(reference=w715, "Value"=w714) -> ()  [unwired: 1 in, 2 out]
        n427 = case shown="错误" w712 {
          tunnel: ["读取成功" ("消息") "读取失败" ("消息")] -> w713
          frame No Error {
          }
          frame Error {
          }
        }
        n428 = One Button Dialog(message=w713) -> ()  [unwired: 1 in, 1 out]
      }
      event "量程切换阈值写入": Value Change {
        n429 = event-data() -> ()  [unwired: 1 in, 6 out]
        n430 = property class="Enum (严格)"(reference=w724) -> ("Value"=w723:enum16{"总磷", "总氮"})  [unwired: 1 in, 2 out]
        n431 = call "总磷总氮量程写入.vi"("量程参数写入"="量程参数读取", "测量参数"=w723) -> ("error out"=w721:errorcluster)  [unwired: 8 in]
        n432 = case shown="无错误" w721 {
          tunnel: ["写入成功" ("消息") "写入失败" ("消息")] -> w722
          frame No Error {
          }
          frame Error {
          }
        }
        n433 = One Button Dialog(message=w722) -> ()  [unwired: 1 in, 1 out]
      }
    }
  }
